vi "Auto Populated Folder Paser.vi"(9 "Item Indent":i32, 11 "path":path) -> (3 "Item List Out":T1(array[cluster]))   [LabVIEW 2020, in "LV Project Items Parser.lvlib"]
doc: "This recursive VI parses the auto-populated folder in disk and lists all elements in it and its subfolders, until it reaches the deepest level in the directory chain."
uses:
  LV Project Items Parser.lvlib
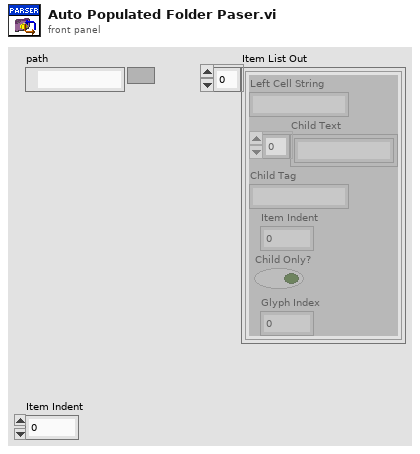
[diagram p1: front panel]
types:
  T1 = cluster{"Left Cell String":string, "Child Text":string[], "Child Tag":string, "Item Indent":i32, "Child Only?":bool, "Glyph Index":i32}[]
  T2 = cluster{"Left Cell String":string, "Child Text":string[], "Child Tag":string, "Item Indent":i32, "Child Only?":bool, "Glyph Index":i32}
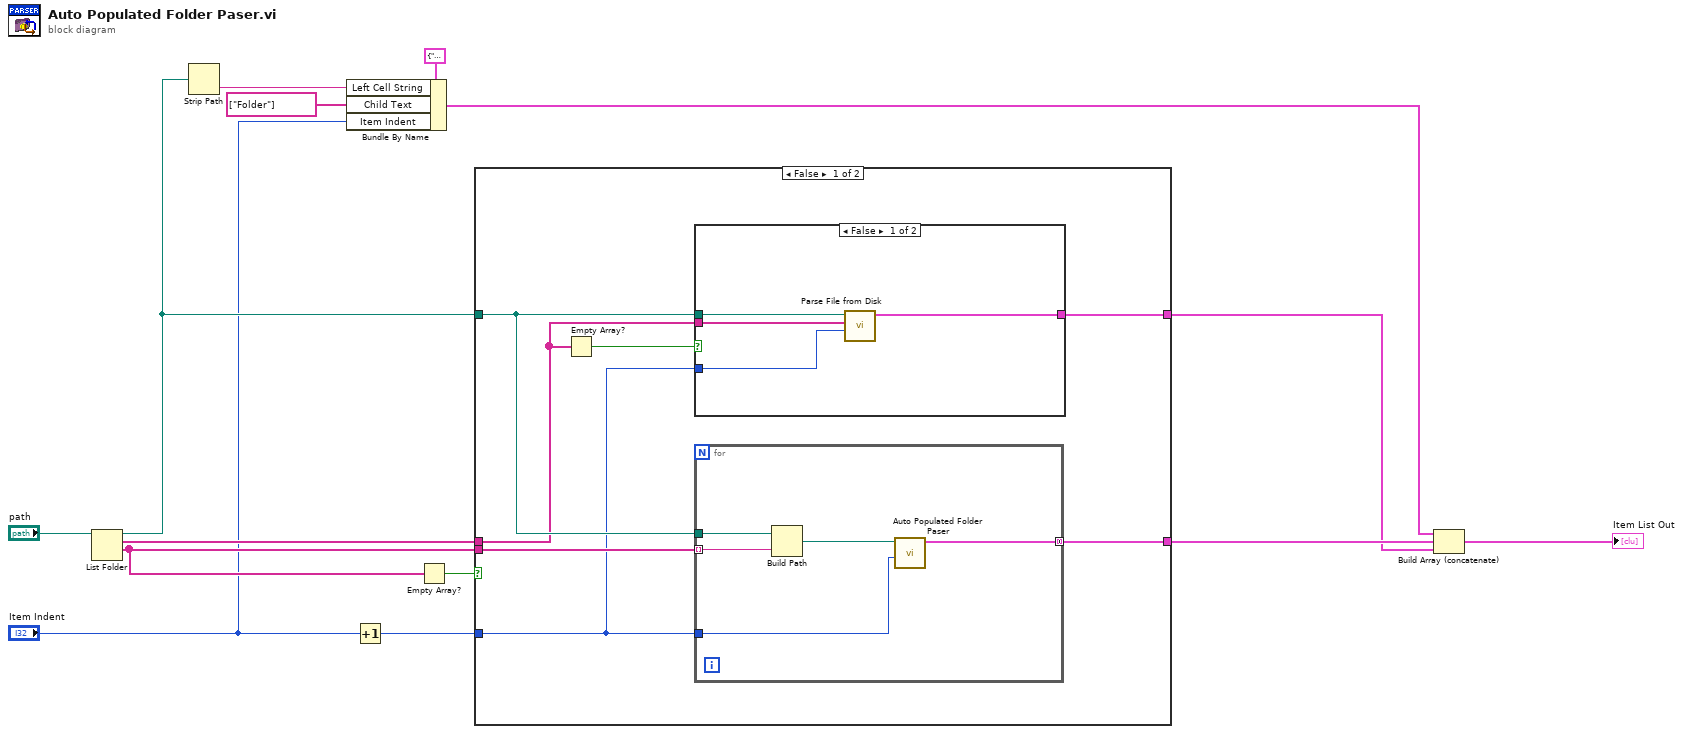
[diagram p0: block diagram]
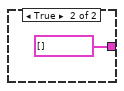
[diagram p2: hidden frame]
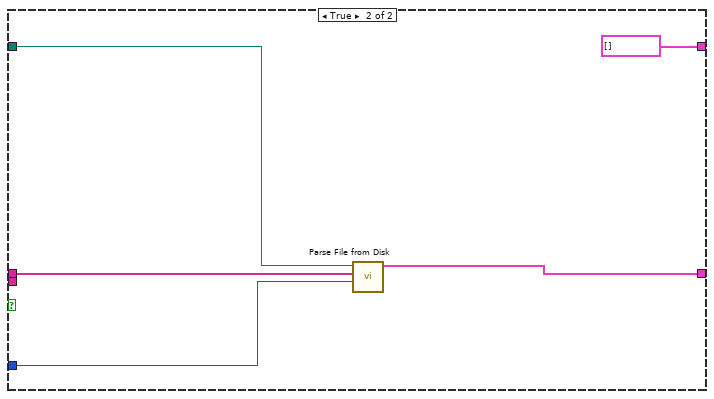
[diagram p3: hidden frame]
diagram:
  n1 = List Folder(path="path") -> (path out=w11:path, filenames=w4:string[], folder names=w12:string[])  [unwired: 3 in, 1 out]
  n2 = Strip Path(path=w11) -> (name=w10:string)  [unwired: 1 out]
  n3 = Bundle By Name(cluster=T2 {"Left Cell String"="", "Child Text"=[], "Child Tag"="", "Item Indent"=0, "Child Only?"=FALSE, "Glyph Index"=0} ("Item"), "Left Cell String"=w10, "Child Text"=string[] ["Folder"], "Item Indent"="Item Indent") -> (w6:T2)
  n4 = Increment(x="Item Indent") -> (x+1=w1:i32)
  n5 = Empty Array?(array=w12) -> (empty?=w5:bool)
  n6 = case shown="False" w5 {
    tunnel: [w20 w36] -> w14
    tunnel: w4 -> [w15 w35]
    tunnel: w1 -> [w16 w34]
    tunnel: w12 -> [w21 _]
    tunnel: w11 -> [w17 w32]
    tunnel: [w19 T1 []] -> w2
    frame False {
      n7 = Empty Array?(array=w15) -> (empty?=w18:bool)
      n8 = case shown="False" w18 {
        tunnel: w15 -> [w23 _]
        tunnel: w16 -> [w22 _]
        tunnel: [w25 T1 []] -> w19
        tunnel: w17 -> [w24 _]
        frame False {
          n9 = call "Parse File from Disk.vi"("Numeric"=w22, "filenames"=w23, "path in"=w24) -> ("Tree Items Array"=w25:T1)  [unwired: 8 in]
        }
        frame True {
        }
      }
      n10 = for {
        tunnel: w21 -> [w31] mode=indexing
        tunnel: [w29] -> w20 mode=concatenating
        tunnel: w16 -> [w28]
        tunnel: w17 -> [w27]
        n11 = Build Path(base path=w27, name or relative path=w31) -> (appended path=w30:path)
        n12 = call "Auto Populated Folder Paser.vi"("Item Indent"=w28, "path"=w30) -> ("Item List Out"=w29:T1)  [unwired: 9 in]
      }
    }
    frame True {
      n13 = call "Parse File from Disk.vi"("Numeric"=w34, "filenames"=w35, "path in"=w32) -> ("Tree Items Array"=w36:T1)  [unwired: 8 in]
    }
  }
  n14 = Build Array (concatenate)(w6, w14, w2) -> (→"Item List Out":T1)
